vi "ChanParam2.vi"(0 "Num.MaxCurrTime":refnum<vi>, 1 "I Max Threshold":refnum<vi>, 2 "I2t":refnum<vi>, 3 "Init":bool, 4 "I Nominal":refnum<vi>, 5 "Group control":refnum<vi>, 6 "Tech.Data":refnum<vi>) -> (20 "Num.MaxCurrTime out":refnum<vi>, 21 "I Max Threshold out":refnum<vi>, 22 "I Nominal out":refnum<vi>, 23 "I2t out":refnum<vi>, 24 "Group control out":refnum<vi>, 25 "Tech.Data out":refnum<vi>)   [LabVIEW 2017]
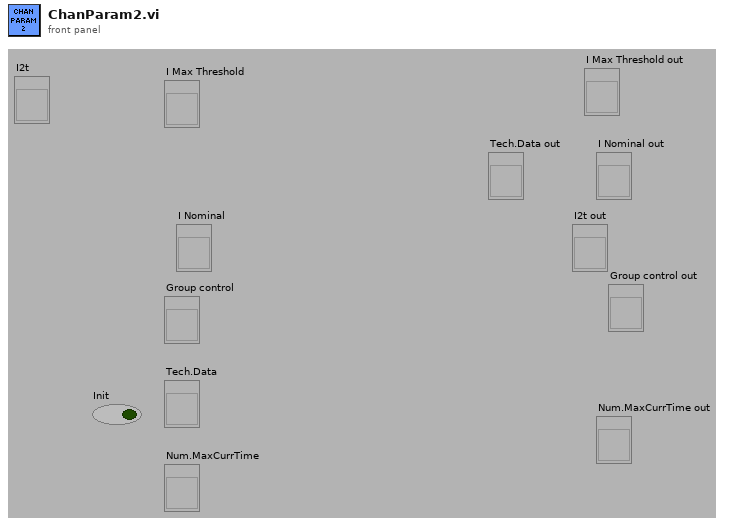
[diagram p1: front panel]
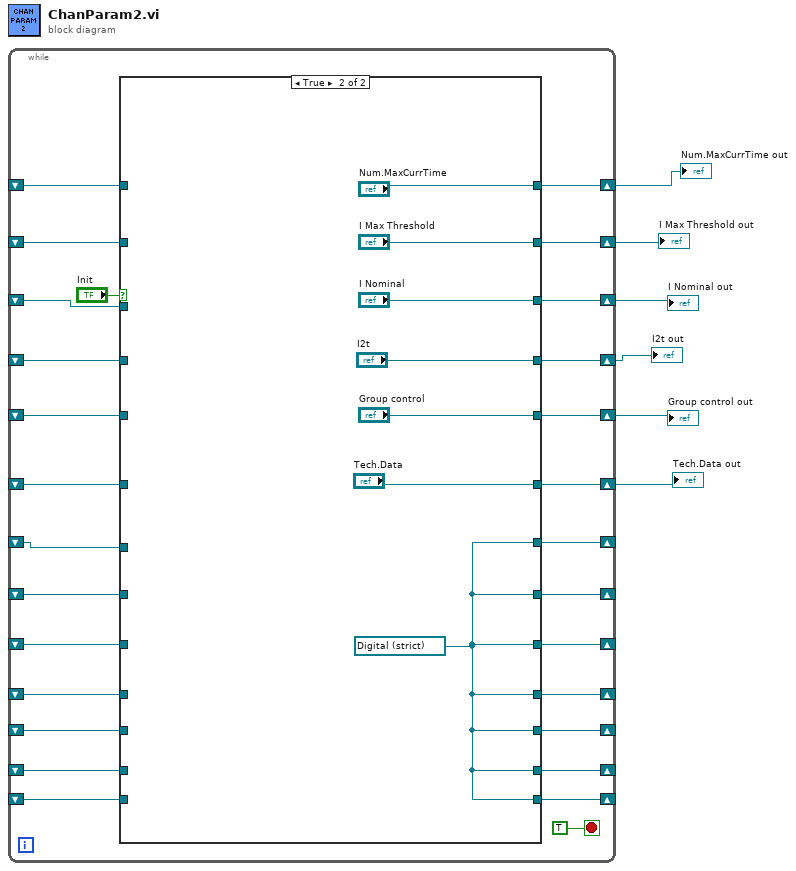
[diagram p0: block diagram]
diagram:
  n1 = while {
    shift-right: [w23] -> w6
    shift-left: _ -> [w29]
    shift-right: [w33] -> w5
    shift-left: _ -> [w28]
    shift-right: [w32] -> w3
    shift-left: _ -> [w27]
    shift-right: [w31] -> w2
    shift-left: _ -> [w26]
    shift-right: [w30] -> w4
    shift-left: _ -> [w25]
    shift-right: [w22] -> w1
    shift-left: _ -> [w21]
    shift-right: [w20] -> _
    shift-left: _ -> [w19]
    shift-right: [w18] -> _
    shift-left: _ -> [w12]
    shift-right: [w17] -> _
    shift-left: _ -> [w11]
    shift-right: [w16] -> _
    shift-left: _ -> [w10]
    shift-right: [w15] -> _
    shift-left: _ -> [w9]
    shift-right: [w14] -> _
    shift-left: _ -> [w8]
    shift-right: [w13] -> _
    shift-left: _ -> [w7]
    stop <- TRUE stop-if-true
    n2 = case shown="True" "Init" {
      tunnel: [w43 "Num.MaxCurrTime"] -> w23
      tunnel: [w47 "I Max Threshold"] -> w33
      tunnel: [w46 "I Nominal"] -> w32
      tunnel: [w45 "I2t"] -> w31
      tunnel: [w44 "Group control"] -> w30
      tunnel: w29 -> [w43 _]
      tunnel: w28 -> [w47 _]
      tunnel: w27 -> [w46 _]
      tunnel: w26 -> [w45 _]
      tunnel: w25 -> [w44 _]
      tunnel: [w42 "Tech.Data"] -> w22
      tunnel: w21 -> [w42 _]
      tunnel: [w41 w52] -> w20
      tunnel: w19 -> [w41 _]
      tunnel: [w40 w52] -> w18
      tunnel: [w39 w52] -> w17
      tunnel: [w38 w52] -> w16
      tunnel: [w37 w52] -> w15
      tunnel: [w36 w52] -> w14
      tunnel: [w35 w52] -> w13
      tunnel: w12 -> [w40 _]
      tunnel: w11 -> [w39 _]
      tunnel: w10 -> [w38 _]
      tunnel: w9 -> [w37 _]
      tunnel: w8 -> [w36 _]
      tunnel: w7 -> [w35 _]
      frame False {
      }
      frame True {
        w52 = refnum<vi> refnum ("Current Threshold in 2")
      }
    }
  }
  "Num.MaxCurrTime out" <- w6
  "I Max Threshold out" <- w5
  "I Nominal out" <- w3
  "Group control out" <- w4
  "I2t out" <- w2
  "Tech.Data out" <- w1
